vi "Tray_main_TrayCtrl.vi"(7 "Enum":T3=enum."TrayDataToUI", 8 "error in":errorcluster, 9 "TrayType":T1, 10 "Index":i32, 11 "TrayRefIn":T4) -> (0 "error Out":errorcluster)   [LabVIEW 2015]
uses:
  subvi/Tray/Tray_TrayCtrl_Action.ctl
  subvi/Tray/Tray_TrayName.ctl
  global/Tray_ArrAndData.vi
panel:
  out "array type (2D Dbl)":T2
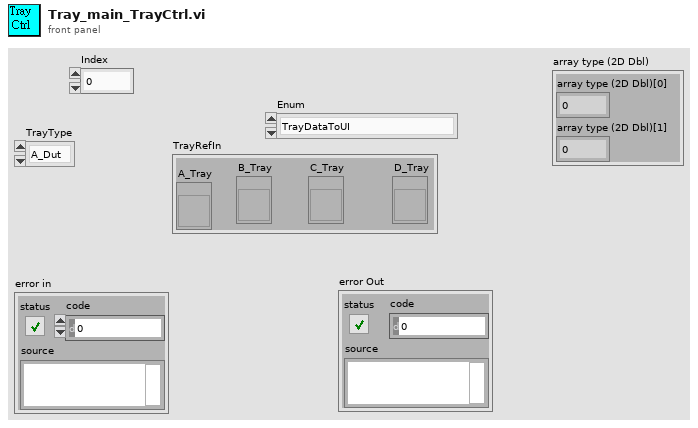
[diagram p1: front panel]
types:
  T1 = typedef "Tray_TrayName.ctl" = enum16{"A_Dut", "B_Pass", "C_NGR", "D_NGL"}
  T2 = cluster{"array type (2D Dbl)[0]":i32, "array type (2D Dbl)[1]":i32}
  T3 = typedef "Tray_TrayCtrl_Action.ctl" = enum16{"InitialTray", "TrayOut", "TrayIn", "SetTray", "TrayDataToUI"}
  T4 = cluster{"A_Tray":refnum<vi>, "B_Tray":refnum<vi>, "C_Tray":refnum<vi>, "D_Tray":refnum<vi>}
  T5 = cluster{"XY_ATray":cluster{"X":i32, "Y":i32}, "Initial color":u32, "FinalColor":u32}
  T6 = cluster{"XY_BTray":cluster{"X":i32, "Y":i32}, "Initial color":u32, "FinalColor":u32}
  T7 = cluster{"XY_CTray":cluster{"X":i32, "Y":i32}, "Initial color":u32, "FinalColor":u32}
  T8 = cluster{"XY_DTray":cluster{"X":i32, "Y":i32}, "Initial color":u32, "FinalColor":u32}
  T9 = typedef "LVPositionTypeDef.ctl" = cluster{"Left":i32, "Top":i32}
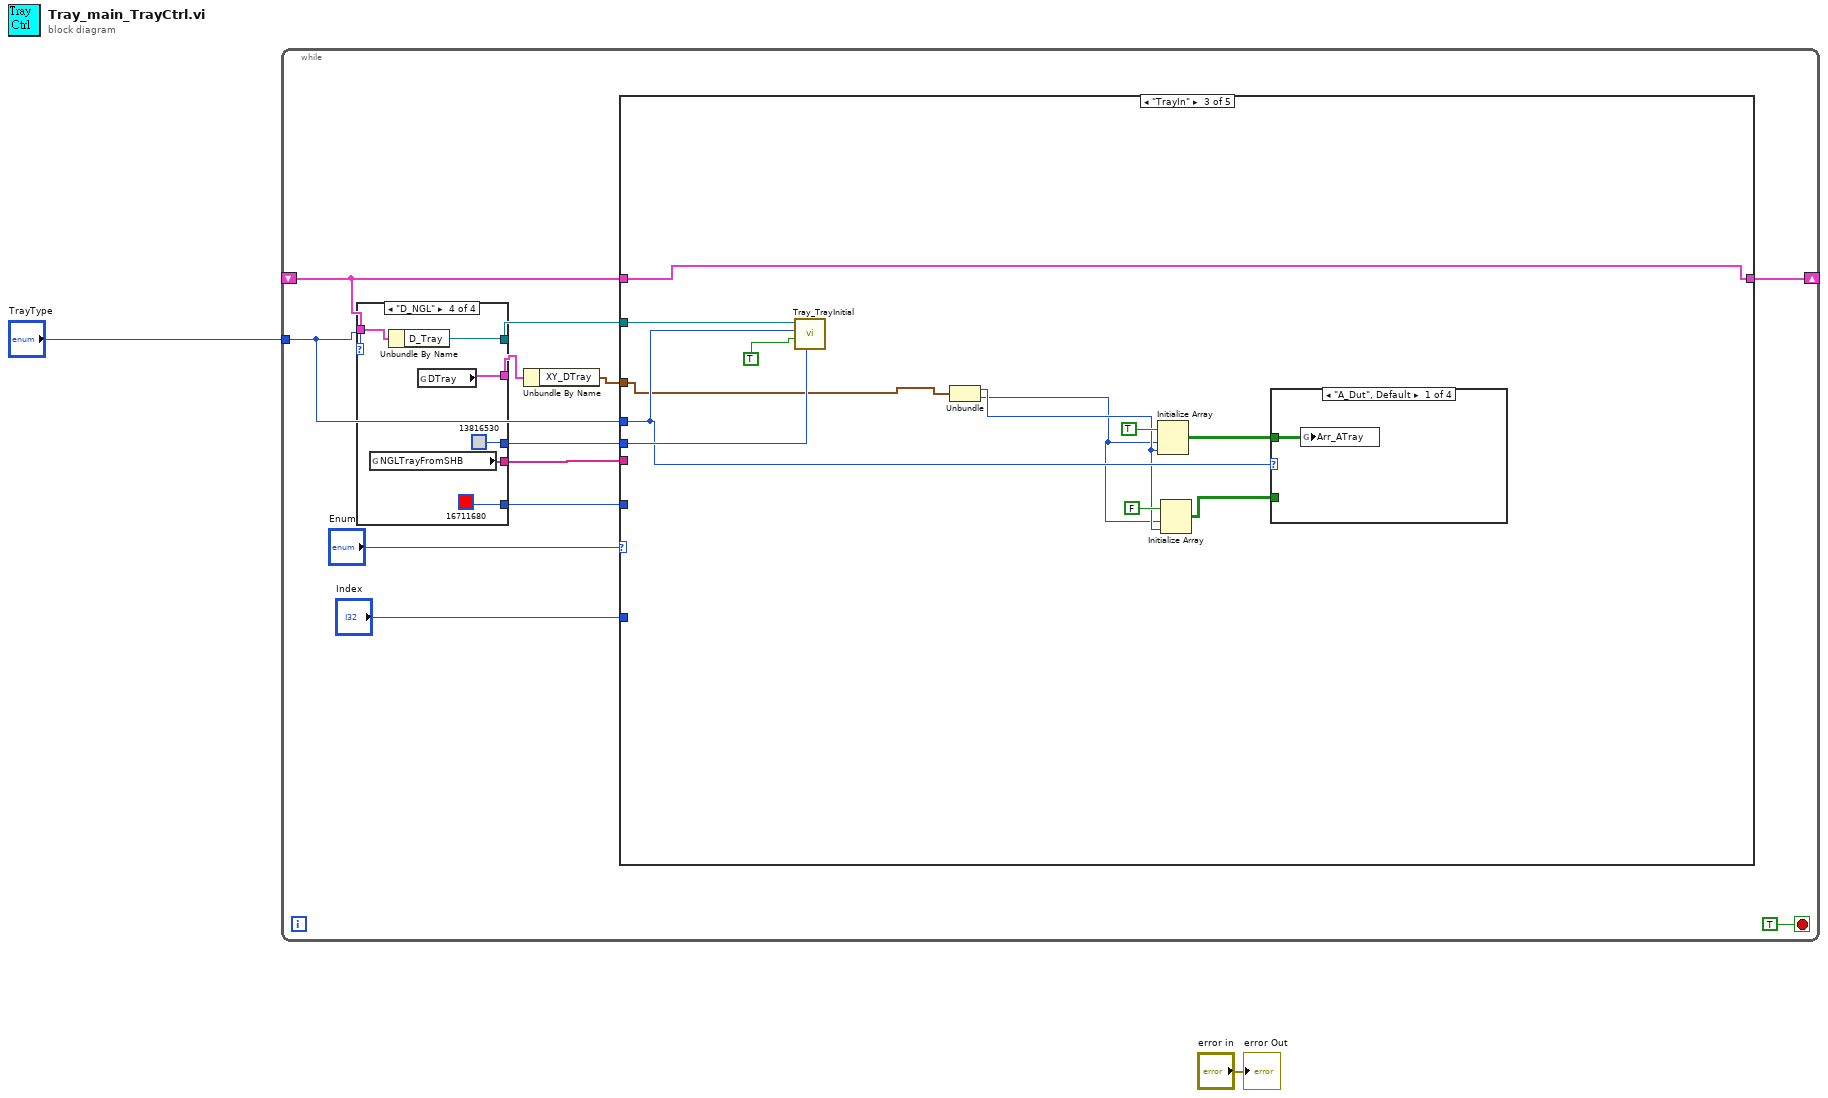
[diagram p0: block diagram]
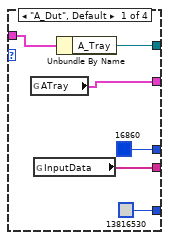
[diagram p2: hidden frame]
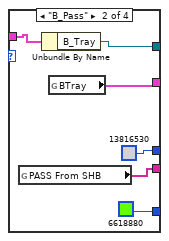
[diagram p3: hidden frame]
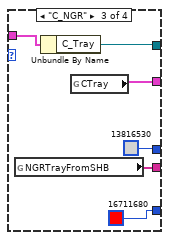
[diagram p4: hidden frame]
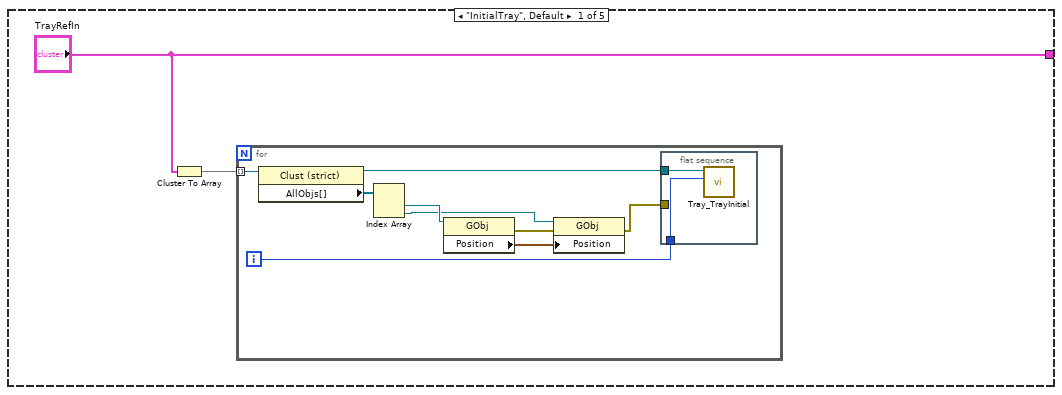
[diagram p5: hidden frame]
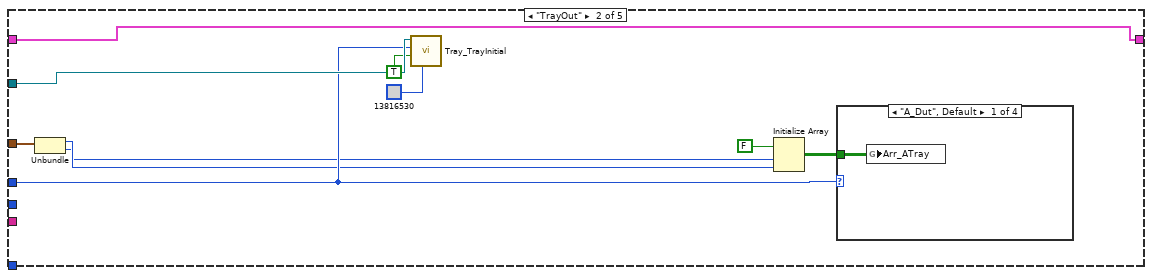
[diagram p6: hidden frame]
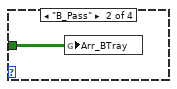
[diagram p7: hidden frame]
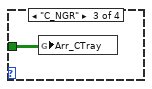
[diagram p8: hidden frame]
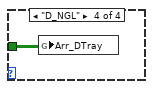
[diagram p9: hidden frame]
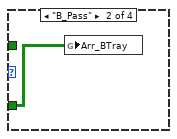
[diagram p10: hidden frame]
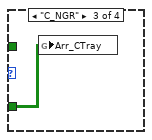
[diagram p11: hidden frame]
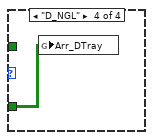
[diagram p12: hidden frame]
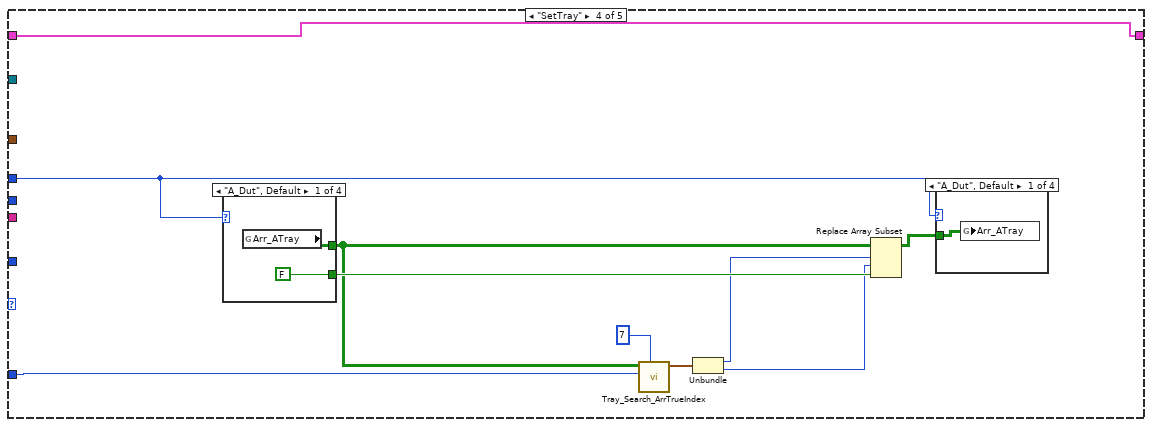
[diagram p13: hidden frame]
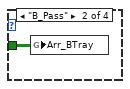
[diagram p14: hidden frame]
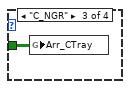
[diagram p15: hidden frame]
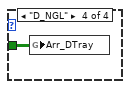
[diagram p16: hidden frame]
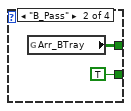
[diagram p17: hidden frame]
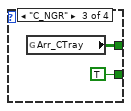
[diagram p18: hidden frame]
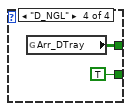
[diagram p19: hidden frame]
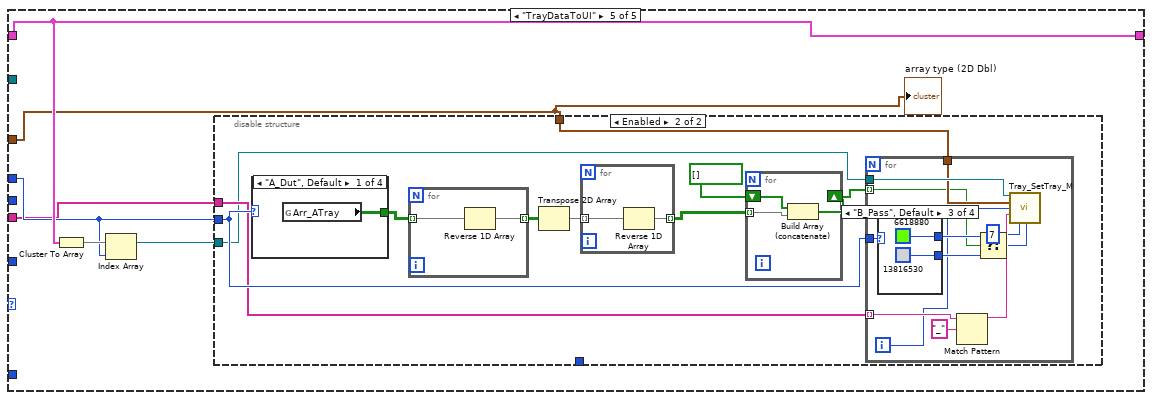
[diagram p20: hidden frame]
diagram:
  n1 = while {
    shift-right: [w14] -> _
    shift-left: _ -> [w11]
    tunnel: "TrayType" -> [w10]
    stop <- TRUE stop-if-true
    n2 = case shown="\"D_NGL\"" w10 {
      tunnel: w11 -> [w20 w26 w32 w38]
      tunnel: [w19 w25 w31 w37] -> w9
      tunnel: [w17 w23 w29 w35] -> w6
      tunnel: [u32 16860 ("Initial color") u32 13816530 ("Initial color") u32 13816530 ("Initial color") u32 13816530 ("Initial color")] -> w8
      tunnel: [w16 w22 w28 w34] -> w4
      tunnel: [u32 13816530 ("Initial color") u32 6618880 ("Initial color") u32 16711680 ("Initial color") u32 16711680 ("Initial color")] -> w3
      frame "A_Dut", Default {
        n3 = global read "Tray_ArrAndData.vi" "ATray"() -> (w17:T5)
        n4 = global read "Tray_ArrAndData.vi" "InputData"() -> (w16:string[])
        n5 = Unbundle By Name(w20) -> ("A_Tray"=w19:refnum<vi>)
      }
      frame "B_Pass" {
        n6 = global read "Tray_ArrAndData.vi" "PASS From SHB"() -> (w22:string[])
        n7 = Unbundle By Name(w26) -> ("B_Tray"=w25:refnum<vi>)
        n8 = global read "Tray_ArrAndData.vi" "BTray"() -> (w23:T6)
      }
      frame "C_NGR" {
        n9 = global read "Tray_ArrAndData.vi" "NGRTrayFromSHB"() -> (w28:string[])
        n10 = Unbundle By Name(w32) -> ("C_Tray"=w31:refnum<vi>)
        n11 = global read "Tray_ArrAndData.vi" "CTray"() -> (w29:T7)
      }
      frame "D_NGL" {
        n12 = global read "Tray_ArrAndData.vi" "NGLTrayFromSHB"() -> (w34:string[])
        n13 = Unbundle By Name(w38) -> ("D_Tray"=w37:refnum<vi>)
        n14 = global read "Tray_ArrAndData.vi" "DTray"() -> (w35:T8)
      }
    }
    n15 = Unbundle By Name(w6) -> ("XY_DTray"=w5:cluster{"X":i32, "Y":i32})
    n16 = case shown="\"TrayIn\"" "Enum" {
      tunnel: ["TrayRefIn" w60 w77 w91 w108] -> w14
      tunnel: w11 -> [_ w60 w77 w91 w108]
      tunnel: "Index" -> [_ _ _ w87 _]
      tunnel: w5 -> [_ w56 w68 _ w104]
      tunnel: w10 -> [_ w57 w71 w83 w106]
      tunnel: w9 -> [_ w58 w75 _ _]
      tunnel: w8 -> [_ _ w73 _ _]
      tunnel: w4 -> [_ _ _ _ w105]
      tunnel: w3 -> [_ _ _ _ _]
      frame "InitialTray", Default {
        n17 = Cluster To Array(cluster="TrayRefIn") -> (array=w40:refnum<vi>[])
        n18 = for {
          tunnel: w40 -> [w49] mode=indexing
          i -> [w41]
          n19 = property class="Clust (strict)"(reference=w49) -> (reference out=w43:refnum<vi>, "AllObjs[]"=w48:refnum<vi>[])  [unwired: 1 in, 1 out]
          n20 = Index Array(array=w48) -> (element #1=w47:refnum<vi>, element #2=w46:refnum<vi>)  [unwired: 2 in]
          n21 = property class="GObj"(reference=w47) -> (error out=w45:errorcluster, "Position"=w44:T9)  [unwired: 1 in, 1 out]
          n22 = property class="GObj"(reference=w46, error in=w45, "Position"=w44) -> (error out=w42:errorcluster)  [unwired: 1 out]
          n23 = flat-sequence {
            tunnel: w43 -> [w51]
            tunnel: w42 -> [_]
            tunnel: w41 -> [w50]
            frame #0 {
              n24 = call "Tray_TrayInitial.vi"("TrayCase"=w50, "TrayIn"=w51) -> ()  [unwired: 9 in, 1 out]
            }
          }
        }
      }
      frame "TrayOut" {
        n25 = Unbundle(w56) -> ("X"=w55:i32, "Y"=w54:i32)
        n26 = call "Tray_TrayInitial.vi"("Initial color"=u32 13816530, "SetColor"=TRUE, "TrayCase"=w57, "TrayIn"=w58) -> ()  [unwired: 7 in, 1 out]
        n27 = Initialize Array(FALSE, w54, w55) -> (w59:bool[][])
        n28 = case shown="\"A_Dut\", Default" w57 {
          tunnel: w59 -> [w62 w63 w64 w65]
          frame "A_Dut", Default {
            n29 = global write "Tray_ArrAndData.vi" "Arr_ATray"(w62) -> ()
          }
          frame "B_Pass" {
            n30 = global write "Tray_ArrAndData.vi" "Arr_BTray"(w63) -> ()
          }
          frame "C_NGR" {
            n31 = global write "Tray_ArrAndData.vi" "Arr_CTray"(w64) -> ()
          }
          frame "D_NGL" {
            n32 = global write "Tray_ArrAndData.vi" "Arr_DTray"(w65) -> ()
          }
        }
      }
      frame "TrayIn" {
        n33 = call "Tray_TrayInitial.vi"("Initial color"=w73, "SetColor"=TRUE, "TrayCase"=w71, "TrayIn"=w75) -> ()  [unwired: 7 in, 1 out]
        n34 = Unbundle(w68) -> ("X"=w67:i32, "Y"=w66:i32)
        n35 = Initialize Array(TRUE, w66, w67) -> (w72:bool[][])
        n36 = Initialize Array(FALSE, w66, w67) -> (w69:bool[][])
        n37 = case shown="\"A_Dut\", Default" w71 {
          tunnel: w72 -> [w78 _ _ _]
          tunnel: w69 -> [_ w79 w80 w81]
          frame "A_Dut", Default {
            n38 = global write "Tray_ArrAndData.vi" "Arr_ATray"(w78) -> ()
          }
          frame "B_Pass" {
            n39 = global write "Tray_ArrAndData.vi" "Arr_BTray"(w79) -> ()
          }
          frame "C_NGR" {
            n40 = global write "Tray_ArrAndData.vi" "Arr_CTray"(w80) -> ()
          }
          frame "D_NGL" {
            n41 = global write "Tray_ArrAndData.vi" "Arr_DTray"(w81) -> ()
          }
        }
      }
      frame "SetTray" {
        n42 = case shown="\"A_Dut\", Default" w83 {
          tunnel: [w97 w99 w101 w103] -> w82
          tunnel: [FALSE TRUE TRUE TRUE] -> w89
          frame "A_Dut", Default {
            n43 = global read "Tray_ArrAndData.vi" "Arr_ATray"() -> (w97:bool[][])
          }
          frame "B_Pass" {
            n44 = global read "Tray_ArrAndData.vi" "Arr_BTray"() -> (w99:bool[][])
          }
          frame "C_NGR" {
            n45 = global read "Tray_ArrAndData.vi" "Arr_CTray"() -> (w101:bool[][])
          }
          frame "D_NGL" {
            n46 = global read "Tray_ArrAndData.vi" "Arr_DTray"() -> (w103:bool[][])
          }
        }
        n47 = call "Tray_Search_ArrTrueIndex.vi"("Direction"=u16 7, "index"=w87, "Input_Arr"=w82) -> ("indexTransXY"=w86:cluster{"Y":i32, "X":i32})  [unwired: 6 in, 2 out]
        n48 = Unbundle(w86) -> ("Y"=w85:i32, "X"=w84:i32)
        n49 = Replace Array Subset(array=w82, new element=w89, index (row)=w85, index (col)=w84) -> (w90:bool[][])
        n50 = case shown="\"A_Dut\", Default" w83 {
          tunnel: w90 -> [w92 w93 w94 w95]
          frame "A_Dut", Default {
            n51 = global write "Tray_ArrAndData.vi" "Arr_ATray"(w92) -> ()
          }
          frame "B_Pass" {
            n52 = global write "Tray_ArrAndData.vi" "Arr_BTray"(w93) -> ()
          }
          frame "C_NGR" {
            n53 = global write "Tray_ArrAndData.vi" "Arr_CTray"(w94) -> ()
          }
          frame "D_NGL" {
            n54 = global write "Tray_ArrAndData.vi" "Arr_DTray"(w95) -> ()
          }
        }
      }
      frame "TrayDataToUI" {
        n55 = Cluster To Array(cluster=w108) -> (array=w109:refnum<vi>[])
        n56 = Index Array(array=w109, index=w106) -> (element=w107:refnum<vi>)
        n57 = disable-structure shown="Enabled" {
          disable-tunnel: w104 -> [w116 w121]
          disable-tunnel: _ -> [w115 _]
          disable-tunnel: w107 -> [w113 w123]
          disable-tunnel: w106 -> [w112 w125]
          disable-tunnel: w105 -> [w110 w124]
          frame Disabled {
            n58 = call "Tray_TrayInitial.vi"("SetColor"=FALSE, "TrayCase"=w112, "TrayIn"=w113) -> ("error Out"=w114:errorcluster)  [unwired: 8 in]
            n59 = call "Tray_TrayDataToUIByNumber.vi"("TrayInRefIn"=w113, "ItemFrom"=w110, "Index"=w115, "TrayType"=w112, "TraySize"=w116, "error in"=w114) -> ()  [unwired: 9 in, 1 out]
          }
          frame Enabled {
            n60 = case shown="\"A_Dut\", Default" w125 {
              tunnel: [w154 w155 w156 w157] -> w117
              frame "A_Dut", Default {
                n61 = global read "Tray_ArrAndData.vi" "Arr_ATray"() -> (w154:bool[][])
              }
              frame "B_Pass" {
                n62 = global read "Tray_ArrAndData.vi" "Arr_BTray"() -> (w155:bool[][])
              }
              frame "C_NGR" {
                n63 = global read "Tray_ArrAndData.vi" "Arr_CTray"() -> (w156:bool[][])
              }
              frame "D_NGL" {
                n64 = global read "Tray_ArrAndData.vi" "Arr_DTray"() -> (w157:bool[][])
              }
            }
            n65 = for {
              tunnel: w117 -> [w128] mode=indexing
              tunnel: [w127] -> w119 mode=indexing
              n66 = Reverse 1D Array(array=w128) -> (reversed array=w127:bool[])
            }
            n67 = Transpose 2D Array(2D array=w119) -> (transposed array=w120:bool[][])
            n68 = for {
              tunnel: w120 -> [w130] mode=indexing
              tunnel: [w129] -> w118 mode=indexing
              n69 = Reverse 1D Array(array=w130) -> (reversed array=w129:bool[])
            }
            n70 = for {
              tunnel: w118 -> [w153] mode=indexing
              shift-right: [w152] -> w122
              shift-left: bool[] [] -> [w151]
              n71 = Build Array (concatenate)(w151, w153) -> (w152:bool[])
            }
            n72 = for {
              tunnel: w125 -> [w136]
              tunnel: w124 -> [w135] mode=indexing
              tunnel: w123 -> [w134]
              tunnel: w121 -> [w133]
              tunnel: w122 -> [w131] mode=indexing
              i -> [w132]
              n73 = case shown="\"B_Pass\", Default" w136 {
                tunnel: [u32 16711680 ("Initial color") u32 16711680 ("Initial color") u32 6618880 ("Initial color") u32 16860 ("Initial color")] -> w138
                tunnel: [u32 13816530 ("Initial color") u32 13816530 ("Initial color") u32 13816530 ("Initial color") u32 13816530 ("Initial color")] -> w139
                frame "C_NGR" {
                }
                frame "D_NGL" {
                }
                frame "B_Pass", Default {
                }
                frame "A_Dut" {
                }
              }
              n74 = Match Pattern(string=w135, regular expression="_") -> (before substring=w142:string)  [unwired: 1 in, 3 out]
              n75 = Select(t=w138, s=w131, f=w139) -> (s? t:f=w140:u32)
              n76 = call "Tray_SetTray_M.vi"("TrayIn"=w134, "GridSize"=w133, "Index Number"=w132, "String"=w142, "Direction"=u16 7, "Color Box"=w140) -> ()  [unwired: 9 in, 1 out]
            }
          }
        }
        "array type (2D Dbl)" <- w104
      }
    }
  }
  "error Out" <- "error in"
